vi "Section Page.vi"(8 "error in (no error)":errorcluster, 11 "Node Ptr":T1 format="%.0x") -> (0 "error out":errorcluster)   [LabVIEW 2019, in "Protection and Counter Addon System Explorer.lvlib"]
uses:
  Protection and Counter Addon System Explorer.lvlib
  <vilib>/NI VeriStand/Custom Device API/Custom Device Item Ref.ctl
  Addon Shared/SubVIs/GUID Lookup.vi
  <vilib>/NI VeriStand/Custom Device API/Custom Device API.lvlib
  Addon Shared/Protection and Counter Addon Shared.lvlib
panel:
  in  "SHDocVw.IWebBrowser2":refnum<k7>(container)
types:
  T1 = typedef "Custom Device API.lvlib/Custom Device Item Ref.ctl" = u64
  T2 = typedef "Custom Device API.lvlib/Custom Device Item Info.ctl" = cluster{"Name":string, "Is Channel":bool, "GUID":string, "Is Waveform":bool}
  T3 = typedef "Custom Device API.lvlib/Custom Device Commands.ctl" = enum16{"Default", "Item renamed", "Shutdown", "Dynamic button pressed"}
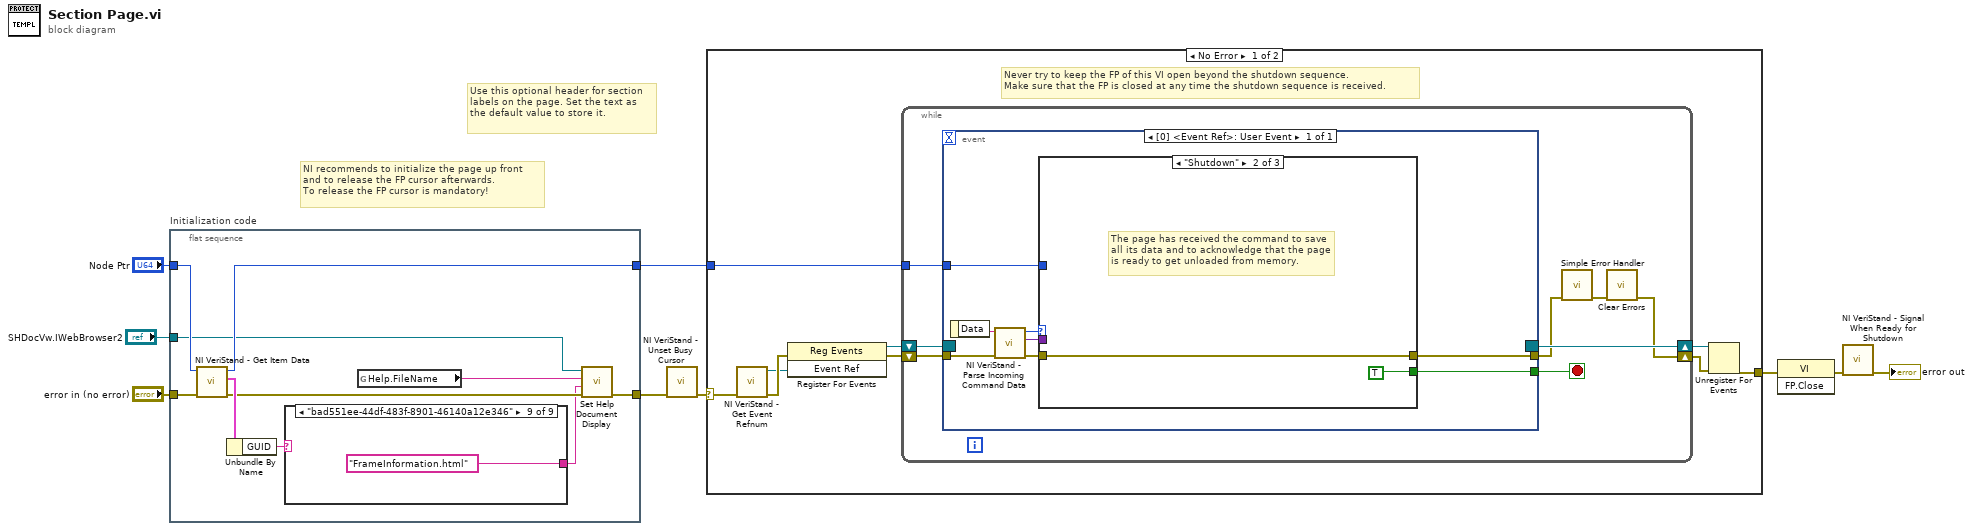
[diagram p0: block diagram]
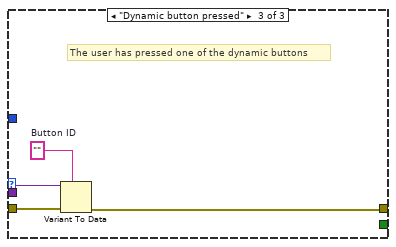
[diagram p3: hidden frame]
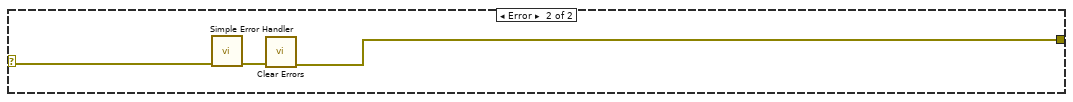
[diagram p4: hidden frame]
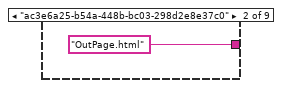
[diagram p6: hidden frame]
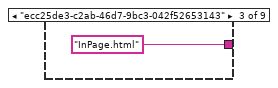
[diagram p7: hidden frame]
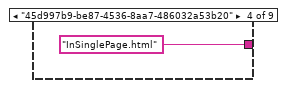
[diagram p8: hidden frame]
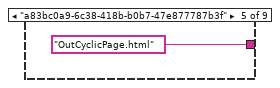
[diagram p9: hidden frame]
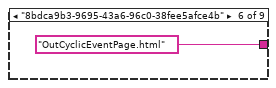
[diagram p10: hidden frame]
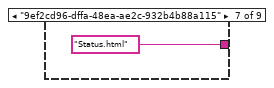
[diagram p11: hidden frame]
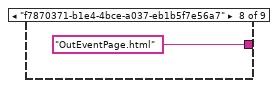
[diagram p12: hidden frame]
diagram:
  # "Use this optional header for section labels on the page. Set the text as the default value to store it."
  # "NI recommends to initialize the page up front\nand to release the FP cursor afterwards.\nTo release the FP cursor is mandatory!"
  n1 = flat-sequence "Initialization code" {
    tunnel: "error in (no error)" -> [w17]
    tunnel: "Node Ptr" -> [w19]
    tunnel: [w13] -> w5
    tunnel: [w18] -> w2
    tunnel: "SHDocVw.IWebBrowser2" -> [w11]
    frame #0 {
      n2 = call <vilib>:"NI VeriStand - Get Item Data.vi"("error in (no error)"=w17, "Item Ref in"=w19) -> ("error out"=w14:errorcluster, "Item Info"=w16:T2, "Item Ref out"=w18:T1)  [unwired: 6 in, 1 out]
      n3 = Unbundle By Name(w16) -> ("GUID"=w15:string)
      n4 = case shown="\"bad551ee-44df-483f-8901-46140a12e346\"" w15 {
        tunnel: [_ "OutPage.html" ("HTML File") "InPage.html" ("HTML File") "InSinglePage.html" ("HTML File") "OutCyclicPage.html" ("HTML File") "OutCyclicEventPage.html" ("HTML File") "Status.html" ("HTML File") "OutEventPage.html" ("HTML File") "FrameInformation.html" ("HTML File")] -> w12
        frame Default {
        }
        frame "ac3e6a25-b54a-448b-bc03-298d2e8e37c0" {
        }
        frame "ecc25de3-c2ab-46d7-9bc3-042f52653143" {
        }
        frame "45d997b9-be87-4536-8aa7-486032a53b20" {
        }
        frame "a83bc0a9-6c38-418b-b0b7-47e877787b3f" {
        }
        frame "8bdca9b3-9695-43a6-96c0-38fee5afce4b" {
        }
        frame "9ef2cd96-dffa-48ea-ae2c-932b4b88a115" {
        }
        frame "f7870371-b1e4-4bce-a037-eb1b5f7e56a7" {
        }
        frame "bad551ee-44df-483f-8901-46140a12e346" {
        }
      }
      n5 = global read "GUID Lookup.vi" "Help.FileName"() -> (w10:string)
      n6 = call "Set Help Document Display.vi"("error in (no error)"=w14, "HTML File"=w12, "Main CHM File"=w10, "SHDocVw.IWebBrowser2"=w11) -> ("error out"=w13:errorcluster)  [unwired: 7 in]
    }
  }
  n7 = call <vilib>:"NI VeriStand - Unset Busy Cursor.vi"("error in (no error)"=w5) -> ("error out"=w4:errorcluster)  [unwired: 10 out]
  n8 = case shown="No Error" w4 {
    selector: w4 -> [w28 w62]
    tunnel: [w33 w60] -> w9
    tunnel: w2 -> [w29 _]
    frame No Error {
      # "Never try to keep the FP of this VI open beyond the shutdown sequence.\nMake sure that the FP is closed at any time the shutdown sequence is received."
      n9 = call <vilib>:"NI VeriStand - Get Event Refnum.vi"("error in (no error)"=w28) -> ("error out"=w36:errorcluster, "Event Ref"=w32:refnum<user-event>)  [unwired: 9 out]
      n10 = register-events(error in=w36, w32) -> (reference out=w30:refnum<event-registration>, error out=w31:errorcluster)  [unwired: 1 in]
      n11 = while {
        tunnel: w29 -> [w40]
        shift-right: [w37] -> w34
        shift-left: w31 -> [w43]
        shift-right: [w44] -> w35
        shift-left: w30 -> [w42]
        stop <- w41 stop-if-true
        n12 = event shown="[0] <Event Ref>: User Event" {
          selector: w42 -> [_]
          dyn-events: [_] -> w44
          timeout: _ -> [_]
          tunnel: w43 -> [w52]
          tunnel: [w48] -> w41
          tunnel: [w47] -> w39
          tunnel: w40 -> [w46]
          event User Event {
            n13 = event-data() -> ("Data"=w51:string)  [unwired: 1 out]
            n14 = call <vilib>:"NI VeriStand - Parse Incoming Command Data.vi"("error in (no error)"=w52, "Incoming data"=w51) -> ("error out"=w50:errorcluster, "Outgoing data"=w45:variant, "Action"=w49:T3)  [unwired: 7 out]
            n15 = case shown="\"Shutdown\"" w49 {
              tunnel: w50 -> [w53 w54 w59]
              tunnel: [_ TRUE _] -> w48
              tunnel: [w53 w54 w56] -> w47
              tunnel: w46 -> [_ _ _]
              tunnel: w45 -> [_ _ w58]
              frame "Default", Default {
              }
              frame "Shutdown" {
                # "The page has received the command to save all its data and to acknowledge that the page is ready to get unloaded from memory."
              }
              frame "Dynamic button pressed" {
                w57 = ""  # Button ID
                # "The user has pressed one of the dynamic buttons"
                n16 = Variant To Data(error in=w59, type=w57, Variant=w58) -> (error out=w56:errorcluster)  [unwired: 1 out]
              }
            }
          }
        }
        n17 = call <vilib>:"Simple Error Handler.vi"("error in (no error)"=w39) -> ("error out"=w38:errorcluster)  [unwired: 1 in, 7 out]
        n18 = call <vilib>:"Clear Errors.vi"("error in (no error)"=w38) -> ("error out"=w37:errorcluster)  [unwired: 1 in, 5 out]
      }
      n19 = Unregister For Events(event registration refnum=w35, error in=w34) -> (error out=w33:errorcluster)
    }
    frame Error {
      n20 = call <vilib>:"Simple Error Handler.vi"("error in (no error)"=w62) -> ("error out"=w61:errorcluster)  [unwired: 1 in, 7 out]
      n21 = call <vilib>:"Clear Errors.vi"("error in (no error)"=w61) -> ("error out"=w60:errorcluster)  [unwired: 1 in, 5 out]
    }
  }
  n22 = invoke class="VI" method="FP.Close"(error in=w9) -> (error out=w8:errorcluster)  [unwired: 2 in, 2 out]
  n23 = call <vilib>:"NI VeriStand - Signal When Ready for Shutdown.vi"("error in (no error)"=w8) -> ("error out"=→"error out":errorcluster)  [unwired: 10 out]
